vi "Reset Supply.vi"(8 "error in":errorcluster, 11 "69X_79X in":refnum<class "6972A.lvclass">) -> (0 "error out":errorcluster, 3 "69X_79X out":refnum<class "6972A.lvclass">)   [LabVIEW 2019, in "6972A.lvlib" / "6972A.lvclass"]
uses:
  Library/6972A.lvclass
  Library/6972A.lvclass/6972A.ctl
  builds/Instruments/PowerSupply.lvlibp/Library/PowerSupply.lvclass
  <instrlib>/Agilent N6900 N7900 Series/Agilent N6900 N7900 Series.lvlib
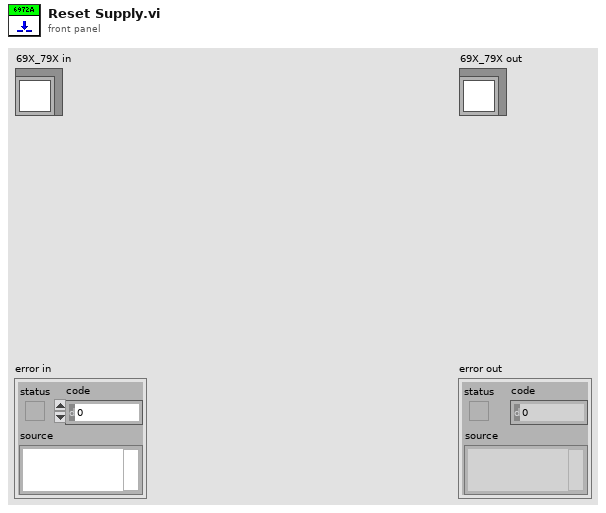
[diagram p1: front panel]
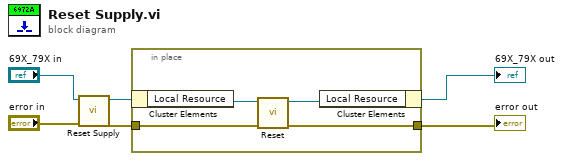
[diagram p0: block diagram]
diagram:
  n1 = call-parent "Reset Supply.vi"("error in"="error in", "PowerSupply in"="69X_79X in") -> ("error out"=w2:errorcluster, "PowerSupply out"=w4:refnum<class "6972A.lvclass">)  [unwired: 8 in]
  n2 = in-place {
    in-place-border: w2 -> [w8]
    in-place-border: [w7] -> w1
    n3 = in-place-cluster #1(w4) -> ("Local Resource"=w10:refnum<visa-resource-name>)
    n4 = call <instrlib>:"Reset.vi"("error in (no error)"=w8, "VISA resource name"=w10) -> ("error out"=w7:errorcluster, "VISA resource name out"=w9:refnum<visa-resource-name>)  [unwired: 8 in]
    n5 = in-place-cluster #1("Local Resource"=w9) -> (→"69X_79X out":refnum<class "6972A.lvclass">)
  }
  "error out" <- w1
